vi "Read Menu  Panel.vi"(8 "error in (no error)":errorcluster, 11 "Interface with menu in":refnum<class "Interface with menu.lvclass">) -> (0 "error out":errorcluster, 2 "Menu  Panel":refnum<vi>, 3 "Interface with menu out":refnum<class "Interface with menu.lvclass">)   [LabVIEW 2015, in "Interface with menu.lvclass"]
uses:
  Interface with menu.lvclass
  Interface with menu.lvclass/Interface with menu.ctl
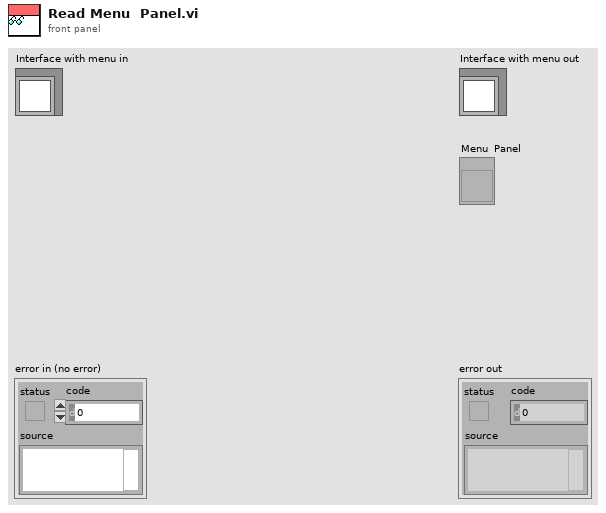
[diagram p1: front panel]
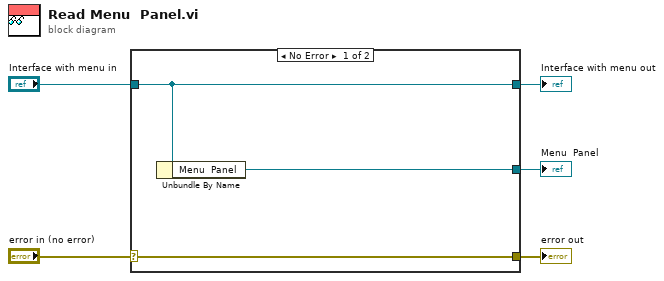
[diagram p0: block diagram]
diagram:
  n1 = case shown="No Error" "error in (no error)" {
    selector: "error in (no error)" -> [w8 w9]
    tunnel: [w8 w9] -> w4
    tunnel: [w7 w10] -> w2
    tunnel: "Interface with menu in" -> [w7 w10]
    tunnel: [w6 _] -> w1
    frame No Error {
      n2 = Unbundle By Name(w7) -> ("Menu  Panel"=w6:refnum<vi>)
    }
    frame Error {
    }
  }
  "error out" <- w4
  "Interface with menu out" <- w2
  "Menu  Panel" <- w1
